vi "Add Remove Test.vi"() -> (0 "error out":errorcluster, 2 "Success Delete":bool, 3 "Success ADD":bool)   [LabVIEW 2015, in "Increment tests.lvlib"]
doc: "Tests the Add Line and Remove Line functions."
uses:
  Increment tests.lvlib
  module/configuration/Increment configuration.lvclass
panel:
  out "Deleted Line":string
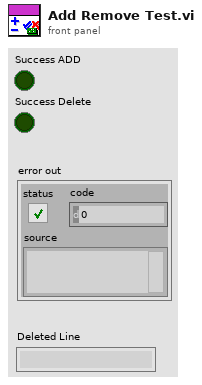
[diagram p1: front panel]
types:
  T1 = typedef "Increment configuration.lvclass/Line.ctl" = cluster{"Name":string, "channel in":refnum<class "TBM channel.lvclass">, "channel out":refnum<class "TBM channel.lvclass">}
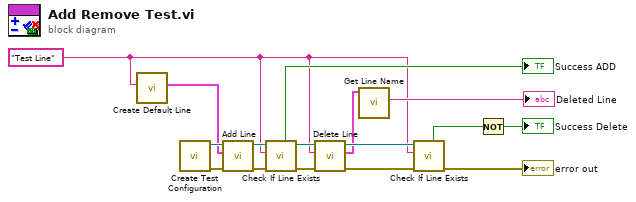
[diagram p0: block diagram]
diagram:
  w1 = "Test Line" ("channel name")
  n1 = call "Create Default Line.vi"("Line Name"=w1) -> ("output cluster"=w2:T1)  [unwired: 10 in]
  n2 = call "Create Test Configuration.vi"() -> ("error out"=w10:errorcluster, "Module Configuration"=w16:refnum<class "Increment configuration.lvclass">)  [unwired: 6 in, 4 out]
  n3 = call "Add Line.vi"("error in"=w10, "Line"=w2, "Increment configuration in"=w16) -> ("error out"=w12:errorcluster, "Increment configuration out"=w15:refnum<class "Increment configuration.lvclass">)  [unwired: 6 in, 1 out]
  n4 = call-dynamic "Check If Line Exists.vi"("error in"=w12, "Name to Locate"=w1, "Increment configuration in"=w15) -> ("error out"=w11:errorcluster, "Increment configuration out"=w14:refnum<class "Increment configuration.lvclass">, "Found?"=→"Success ADD":bool)  [unwired: 4 in, 2 out]
  n5 = call "Delete Line.vi"("error in"=w11, "Line Name"=w1, "Increment configuration in"=w14) -> ("error out"=w9:errorcluster, "Deleted Line"=w4:T1, "Increment configuration out"=w7:refnum<class "Increment configuration.lvclass">)  [unwired: 6 in]
  n6 = call "Get Line Name.vi"("Line in"=w4) -> ("Name"=→"Deleted Line":string)  [unwired: 8 in, 2 out]
  n7 = call-dynamic "Check If Line Exists.vi"("error in"=w9, "Name to Locate"=w1, "Increment configuration in"=w7) -> ("error out"=→"error out":errorcluster, "Found?"=w6:bool)  [unwired: 4 in, 3 out]
  n8 = Not(x=w6) -> (.not. x?=→"Success Delete":bool)
